vi "Receive SGL Value Msg.vi"(8 "error in (no error)":errorcluster, 10 "SGLValueMsg":refnum<class "SGLValueMsg.lvclass">, 11 "IModel in":refnum<class "IModel.lvclass">) -> (0 "error out":errorcluster, 3 "IModel out":refnum<class "IModel.lvclass">)   [LabVIEW 2015, in "IModel.lvlib" / "IModel.lvclass"]
uses:
  IModel.lvclass
  AutoRegistration/ActorAutoRegistration Messages/SGLValueMsg/SGLValueMsg.lvclass
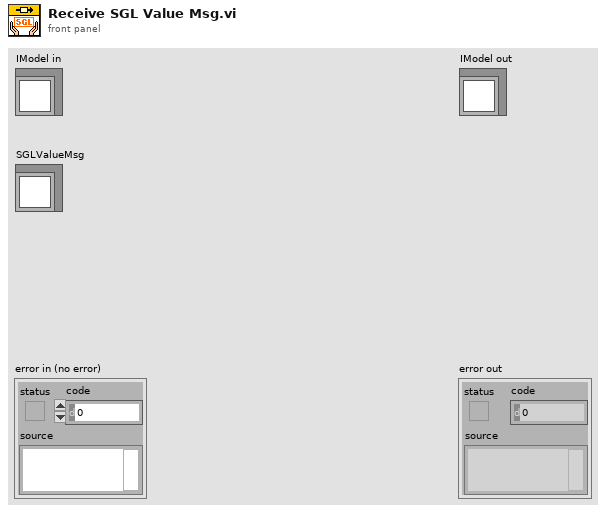
[diagram p1: front panel]
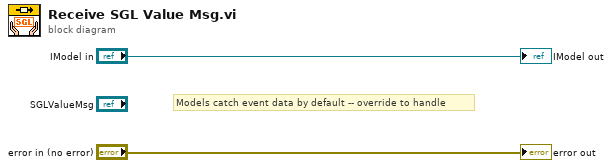
[diagram p0: block diagram]
diagram:
  # "Models catch event data by default -- override to handle"
  "error out" <- "error in (no error)"
  "IModel out" <- "IModel in"
